vi "test_read-nmea-data2.vi"() -> ()   [LabVIEW 2019] (continued)
A,3,85,70,71,84,,,,,,,,,1.18,0.66,0.97,2*04\n\t\n15:14:01.34\tF9P\t$GNGSA,A,3,36,19,11,04,09,12,,,,,,,1.18,0.66,0.97,3*06\n\t\n15:14:01.36\tF9P\t$GNGSA,A,3,14,11,33,,,,,,,,,,1.18,0.66,0.97,4*07\n\t\n15:14:01.38\tF9P\t$GPGSV,3,1,09,02,55,320,27,04,17,043,32,05,38,248,30,06,64,050,27,1*6A\n\t\n15:14:01.40\tF9P\t$GPGSV,3,2,09,09,44,073,35,12,23,276,23,17,32,154,33,19,51,157,29,1*64\n\t\n15:14:01.42\tF9P\t$GPGSV,3,3,09,25,12,306,16,1*5B\n\t\n15:14:01.44\tF9P\t$GPGSV,3,1,09,02,55,320,,04,17,043,21,05,38,248,17,06,64,050,24,6*6C\n\t\n15:14:01.46\tF9P\t$GPGSV,3,2,09,09,44,073,29,12,23,276,13,17,32,154,19,19,51,157,,6*6E\n\t\n15:14:01.48\tF9P\t$GPGSV,3,3,09,25,12,306,,6*5B\n\t\n15:14:01.50\tF9P\t$GLGSV,2,1,08,69,11,031,34,70,70,038,25,71,53,206,26,72,05,210,,1*76\n\t\n15:14:01.52\tF9P\t$GLGSV,2,2,08,77,01,325,,84,19,123,17,85,70,070,29,86,37,330,,1*7B\n\t\n15:14:01.54\tF9P\t$GLGSV,2,1,08,69,11,031,29,70,70,038,,71,53,206,23,72,05,210,,3*7A\n\t\n15:14:01.56\tF9P\t$GLGSV,2,2,08,77,01,325,,84,19,123,23,85,70,070,22,86,37,330,,3*75\n\t\n15:14:01.58\tF9P\t$GAGSV,2,1,08,02,08,296,16,04,67,115,35,09,33,193,22,11,72,001,24,7*7E\n\t\n15:14:01.60\tF9P\t$GAGSV,2,2,08,12,39,103,24,19,25,045,22,25,09,249,,36,26,308,10,7*72\n\t\n15:14:01.62\tF9P\t$GAGSV,2,1,08,02,08,296,,04,67,115,26,09,33,193,,11,72,001,,2*78\n\t\n15:14:01.64\tF9P\t$GAGSV,2,2,08,12,39,103,,19,25,045,,25,09,249,,36,26,308,,2*70\n\t\n15:14:01.66\tF9P\t$GBGSV,1,1,04,11,49,132,27,14,87,114,32,28,,,30,33,61,220,33,1*4B\n\t\n15:14:01.68\tF9P\t$GBGSV,1,1,04,08,,,36,11,49,132,26,14,87,114,28,33,61,220,,3*47\n\t\n15:14:01.70\tF9P\t$GNGLL,3723.58118,N,12656.98443,E,061403.00,A,A*73\n\t\n15:14:01.72\tF9P\t\t\n15:14:01.74\tF9P\t\t\n15:14:01.76\tF9P\t\t\n15:14:01.78\tF9P\t\t\n15:14:01.80\tF9P\t\t\n15:14:01.82\tF9P\t\t\n15:14:01.84\tF9P\t\t\n15:14:01.86\tF9P\t\t\n15:14:01.88\tF9P\t\t\n15:14:01.90\tF9P\t\t\n15:14:01.92\tF9P\t\t\n15:14:01.94\tF9P\t\t\n15:14:01.96\tF9P\t\t\n15:14:01.98\tF9P\t\t\n15:14:02.00\tF9P\t\t\n15:14:02.02\tF9P\t\t\n15:14:02.04\tF9P\t\t\n15:14:02.06\tF9P\t\t\n15:14:02.08\tF9P\t\t\n15:14:02.10\tF9P\t\t\n15:14:02.12\tF9P\t\t\n15:14:02.14\tF9P\t\t\n15:14:02.16\tF9P\t\t\n15:14:02.18\tF9P\t\t\n15:14:02.20\tF9P\t\t\n15:14:02.22\tF9P\t\t\n15:14:02.24\tF9P\t$GNRMC,061404.00,A,3723.58195,N,12656.98403,E,2.222,333.91,250720,,,A,V*01\n\t\n15:14:02.26\tF9P\t$GNVTG,333.91,T,,M,2.222,N,4.115,K,A*29\n\t\n15:14:02.28\tF9P\t$GNGGA,061404.00,3723.58195,N,12656.98403,E,1,12,0.71,48.3,M,18.5,M,,*76\n\t\n15:14:02.30\tF9P\t$GNGSA,A,3,12,06,19,05,17,09,04,02,,,,,1.27,0.71,1.05,1*06\n\t\n15:14:02.32\tF9P\t$GNGSA,A,3,85,70,71,84,,,,,,,,,1.27,0.71,1.05,2*04\n\t\n15:14:02.34\tF9P\t$GNGSA,A,3,36,19,11,04,09,12,,,,,,,1.27,0.71,1.05,3*06\n\t\n15:14:02.36\tF9P\t$GNGSA,A,3,14,11,33,,,,,,,,,,1.27,0.71,1.05,4*07\n\t\n15:14:02.38\tF9P\t$GPGSV,3,1,09,02,55,320,31,04,17,043,35,05,38,248,36,06,64,050,28,1*63\n\t\n15:14:02.40\tF9P\t$GPGSV,3,2,09,09,44,073,35,12,23,276,22,17,32,154,39,19,51,157,33,1*64\n\t\n15:14:02.42\tF9P\t$GPGSV,3,3,09,25,12,306,14,1*59\n\t\n15:14:02.44\tF9P\t$GPGSV,3,1,09,02,55,320,,04,17,043,21,05,38,248,20,06,64,050,23,6*6F\n\t\n15:14:02.46\tF9P\t$GPGSV,3,2,09,09,44,073,21,12,23,276,10,17,32,154,19,19,51,157,,6*65\n\t\n15:14:02.48\tF9P\t$GPGSV,3,3,09,25,12,306,,6*5B\n\t\n15:14:02.50\tF9P\t$GLGSV,2,1,08,69,11,031,34,70,70,038,23,71,53,206,31,72,05,210,,1*76\n\t\n15:14:02.52\tF9P\t$GLGSV,2,2,08,77,01,325,,84,19,123,19,85,70,070,24,86,37,330,,1*78\n\t\n15:14:02.54\tF9P\t$GLGSV,2,1,08,69,11,031,29,70,70,038,,71,53,206,29,72,05,210,,3*70\n\t\n15:14:02.56\tF9P\t$GLGSV,2,2,08,77,01,325,,84,19,123,30,85,70,070,21,86,37,330,,3*74\n\t\n15:14:02.58\tF9P\t$GAGSV,2,1,08,02,08,296,10,04,67,115,32,09,33,193,23,11,72,001,25,7*7F\n\t\n15:14:02.60\tF9P\t$GAGSV,2,2,08,12,39,103,34,19,25,045,30,25,09,249,,36,26,308,13,7*73\n\t\n15:14:02.62\tF9P\t$GAGSV,2,1,08,02,08,296,,04,67,115,32,09,33,193,,11,72,001,,2*7D\n\t\n15:14:02.64\tF9P\t$GAGSV,2,2,08,12,39,103,,19,25,045,,25,09,249,,36,26,308,,2*70\n\t\n15:14:02.66\tF9P\t$GBGSV,1,1,04,11,49,132,33,14,87,114,29,28,,,29,33,61,220,37,1*48\n\t\n15:14:02.68\tF9P\t$GBGSV,1,1,04,08,,,27,11,49,132,29,14,87,114,28,33,61,220,,3*48\n\t\n15:14:02.70\tF9P\t$GNGLL,3723.58195,N,12656.98403,E,061404.00,A,A*75\n\t\n15:14:02.72\tF9P\t\t\n15:14:02.74\tF9P\t\t\n15:14:02.76\tF9P\t\t\n15:14:02.78\tF9P\t\t\n15:14:02.80\tF9P\t\t\n15:14:02.82\tF9P\t\t\n15:14:02.84\tF9P\t\t\n15:14:02.86\tF9P\t\t\n15:14:02.88\tF9P\t\t\n15:14:02.90\tF9P\t\t\n15:14:02.92\tF9P\t\t\n15:14:02.94\tF9P\t\t\n15:14:02.96\tF9P\t\t\n15:14:02.98\tF9P\t\t\n15:14:03.00\tF9P\t\t\n15:14:03.02\tF9P\t\t\n15:14:03.04\tF9P\t\t\n15:14:03.06\tF9P\t\t\n15:14:03.08\tF9P\t\t\n15:14:03.10\tF9P\t\t\n15:14:03.12\tF9P\t\t\n15:14:03.14\tF9P\t\t\n15:14:03.16\tF9P\t\t\n15:14:03.18\tF9P\t\t\n15:14:03.20\tF9P\t\t\n15:14:03.22\tF9P\t\t\n15:14:03.24\tF9P\t$GNRMC,061405.00,A,3723.58265,N,12656.98422,E,1.873,346.43,250720,,,A,V*0F\n\t\n15:14:03.26\tF9P\t$GNVTG,346.43,T,,M,1.873,N,3.469,K,A*20\n\t\n15:14:03.28\tF9P\t$GNGGA,061405.00,3723.58265,N,12656.98422,E,1,12,0.71,47.7,M,18.5,M,,*73\n\t\n15:14:03.30\tF9P\t$GNGSA,A,3,12,06,19,05,17,09,04,02,,,,,1.27,0.71,1.05,1*06\n\t\n15:14:03.32\tF9P\t$GNGSA,A,3,85,70,71,84,,,,,,,,,1.27,0.71,1.05,2*04\n\t\n15:14:03.34\tF9P\t$GNGSA,A,3,36,19,11,04,09,12,,,,,,,1.27,0.71,1.05,3*06\n\t\n15:14:03.36\tF9P\t$GNGSA,A,3,14,11,33,,,,,,,,,,1.27,0.71,1.05,4*07\n\t\n15:14:03.38\tF9P\t$GPGSV,3,1,09,02,55,320,31,04,17,043,32,05,38,248,26,06,64,050,36,1*6A\n\t\n15:14:03.40\tF9P\t$GPGSV,3,2,09,09,44,073,40,12,23,276,21,17,32,154,33,19,51,157,32,1*6E\n\t\n15:14:03.42\tF9P\t$GPGSV,3,3,09,25,12,306,10,1*5D\n\t\n15:14:03.44\tF9P\t$GPGSV,3,1,09,02,55,320,,04,17,043,29,05,38,248,21,06,64,050,29,6*6C\n\t\n15:14:03.46\tF9P\t$GPGSV,3,2,09,09,44,073,30,12,23,276,,17,32,154,21,19,51,157,,6*6F\n\t\n15:14:03.48\tF9P\t$GPGSV,3,3,09,25,12,306,,6*5B\n\t\n15:14:03.50\tF9P\t$GLGSV,2,1,08,69,11,031,35,70,70,038,21,71,53,206,39,72,05,210,,1*7D\n\t\n15:14:03.52\tF9P\t$GLGSV,2,2,08,77,01,325,,84,19,123,29,85,70,070,29,86,37,330,,1*76\n\t\n15:14:03.54\tF9P\t$GLGSV,2,1,08,69,11,031,22,70,70,038,,71,53,206,29,72,05,210,,3*7B\n\t\n15:14:03.56\tF9P\t$GLGSV,2,2,08,77,01,325,,84,19,123,29,85,70,070,21,86,37,330,,3*7C\n\t\n15:14:03.58\tF9P\t$GAGSV,2,1,08,02,08,296,16,04,67,115,29,09,33,193,22,11,72,001,26,7*71\n\t\n15:14:03.60\tF9P\t$GAGSV,2,2,08,12,39,103,29,19,25,045,29,25,08,248,,36,26,308,14,7*70\n\t\n15:14:03.62\tF9P\t$GAGSV,2,1,08,02,08,296,,04,67,115,25,09,33,193,,11,72,001,,2*7B\n\t\n15:14:03.64\tF9P\t$GAGSV,2,2,08,12,39,103,,19,25,045,,25,08,248,,36,26,308,,2*70\n\t\n15:14:03.66\tF9P\t$GBGSV,1,1,04,11,49,132,31,14,87,114,30,28,,,33,33,61,220,29,1*46\n\t\n15:14:03.68\tF9P\t$GBGSV,1,1,04,08,,,28,11,49,132,38,14,87,114,33,33,61,220,,3*4D\n\t\n15:14:03.70\tF9P\t$GNGLL,3723.58265,N,12656.98422,E,061405.00,A,A*7B\n\t\n15:14:03.72\tF9P\t\t\n15:14:03.74\tF9P\t\t\n15:14:03.76\tF9P\t\t\n15:14:03.78\tF9P\t\t\n15:14:03.80\tF9P\t\t\n15:14:03.82\tF9P\t\t\n15:14:03.84\tF9P\t\t\n15:14:03.86\tF9P\t\t\n15:14:03.88\tF9P\t\t\n15:14:03.90\tF9P\t\t\n15:14:03.92\tF9P\t\t\n15:14:03.94\tF9P\t\t\n15:14:03.96\tF9P\t\t\n15:14:03.98\tF9P\t\t\n15:14:04.00\tF9P\t\t\n15:14:04.02\tF9P\t\t\n15:14:04.04\tF9P\t\t\n15:14:04.06\tF9P\t\t\n15:14:04.08\tF9P\t\t\n15:14:04.10\tF9P\t\t\n15:14:04.12\tF9P\t\t\n15:14:04.14\tF9P\t\t\n15:14:04.16\tF9P\t\t\n15:14:04.18\tF9P\t\t\n15:14:04.20\tF9P\t\t\n15:14:04.22\tF9P\t\t\n15:14:04.24\tF9P\t$GNRMC,061406.00,A,3723.58360,N,12656.98387,E,2.422,350.86,250720,,,A,V*05\n\t\n15:14:04.26\tF9P\t$GNVTG,350.86,T,,M,2.422,N,4.486,K,A*23\n\t\n15:14:04.28\tF9P\t$GNGGA,061406.00,3723.58360,N,12656.98387,E,1,12,0.71,47.4,M,18.5,M,,*7F\n\t\n15:14:04.30\tF9P\t$GNGSA,A,3,12,06,19,05,17,09,04,02,,,,,1.27,0.71,1.05,1*06\n\t\n15:14:04.32\tF9P\t$GNGSA,A,3,85,70,71,84,,,,,,,,,1.27,0.71,1.05,2*04\n\t\n15:14:04.34\tF9P\t$GNGSA,A,3,36,19,11,04,09,12,,,,,,,1.27,0.71,1.05,3*06\n\t\n15:14:04.36\tF9P\t$GNGSA,A,3,14,11,33,,,,,,,,,,1.27,0.71,1.05,4*07\n\t\n15:14:04.38\tF9P\t$GPGSV,3,1,09,02,55,320,29,04,17,043,31,05,38,248,37,06,64,050,29,1*6E\n\t\n15:14:04.40\tF9P\t$GPGSV,3,2,09,09,44,073,31,12,23,276,20,17,32,154,41,19,51,157,30,1*6E\n\t\n15:14:04.42\tF9P\t$GPGSV,3,3,09,25,12,306,12,1*5F\n\t\n15:14:04.44\tF9P\t$GPGSV,3,1,09,02,55,320,,04,17,043,24,05,38,248,20,06,64,050,28,6*61\n\t\n15:14:04.46\tF9P\t$GPGSV,3,2,09,09,44,073,23,12,23,276,,17,32,154,22,19,51,157,,6*6E\n\t\n15:14:04.48\tF9P\t$GPGSV,3,3,09,25,12,306,,6*5B\n\t\n15:14:04.50\tF9P\t$GLGSV,2,1,08,69,11,031,34,70,70,038,23,71,53,206,31,72,05,210,,1*76\n\t\n15:14:04.52\tF9P\t$GLGSV,2,2,08,77,01,325,,84,19,123,29,85,70,070,33,86,37,330,,1*7D\n\t\n15:14:04.54\tF9P\t$GLGSV,2,1,08,69,11,031,24,70,70,038,,71,53,206,23,72,05,210,,3*77\n\t\n15:14:04.56\tF9P\t$GLGSV,2,2,08,77,01,325,,84,19,123,24,85,70,070,22,86,37,330,,3*72\n\t\n15:14:04.58\tF9P\t$GAGSV,2,1,08,02,08,296,14,04,67,115,29,09,33,193,22,11,72,001,26,7*73\n\t\n15:14:04.60\tF9P\t$GAGSV,2,2,08,12,39,103,33,19,25,045,29,25,08,248,,36,26,308,13,7*7C\n\t\n15:14:04.62\tF9P\t$GAGSV,2,1,08,02,08,296,,04,67,115,,09,33,193,,11,72,001,,2*7C\n\t\n15:14:04.64\tF9P\t$GAGSV,2,2,08,12,39,103,,19,25,045,,25,08,248,,36,26,308,,2*70\n\t\n15:14:04.66\tF9P\t$GBGSV,1,1,04,11,49,132,36,14,87,114,34,28,,,30,33,61,220,36,1*48\n\t\n15:14:04.68\tF9P\t$GBGSV,1,1,04,08,,,28,11,49,132,32,14,87,114,32,33,61,220,,3*46\n\t\n15:14:04.70\tF9P\t$GNGLL,3723.58360,N,12656.98387,E,061406.00,A,A*74\n\t\n15:14:04.72\tF9P\t\t\n15:14:04.74\tF9P\t\t\n15:14:04.76\tF9P\t\t\n15:14:04.78\tF9P\t\t\n15:14:04.80\tF9P\t\t\n15:14:04.82\tF9P\t\t\n15:14:04.84\tF9P\t\t\n15:14:04.86\tF9P\t\t\n15:14:04.88\tF9P\t\t\n15:14:04.90\tF9P\t\t\n15:14:04.92\tF9P\t\t\n15:14:04.94\tF9P\t\t\n15:14:04.96\tF9P\t\t\n15:14:04.98\tF9P\t\t\n15:14:05.00\tF9P\t\t\n15:14:05.02\tF9P\t\t\n15:14:05.04\tF9P\t\t\n15:14:05.06\tF9P\t\t\n15:14:05.08\tF9P\t\t\n15:14:05.10\tF9P\t\t\n15:14:05.12\tF9P\t\t\n15:14:05.14\tF9P\t\t\n15:14:05.16\tF9P\t\t\n15:14:05.18\tF9P\t\t\n15:14:05.20\tF9P\t\t\n15:14:05.22\tF9P\t\t\n15:14:05.24\tF9P\t$GNRMC,061407.00,A,3723.58436,N,12656.98343,E,1.577,346.00,250720,,,A,V*03\n\t\n15:14:05.26\tF9P\t$GNVTG,346.00,T,,M,1.577,N,2.920,K,A*2F\n\t\n15:14:05.28\tF9P\t$GNGGA,061407.00,3723.58436,N,12656.98343,E,1,12,0.71,45.6,M,18.5,M,,*72\n\t\n15:14:05.30\tF9P\t$GNGSA,A,3,12,06,19,05,17,09,04,02,,,,,1.27,0.71,1.05,1*06\n\t\n15:14:05.32\tF9P\t$GNGSA,A,3,85,70,71,84,,,,,,,,,1.27,0.71,1.05,2*04\n\t\n15:14:05.34\tF9P\t$GNGSA,A,3,36,19,11,04,09,12,,,,,,,1.27,0.71,1.05,3*06\n\t\n15:14:05.36\tF9P\t$GNGSA,A,3,14,11,33,,,,,,,,,,1.27,0.71,1.05,4*07\n\t\n15:14:05.38\tF9P\t$GPGSV,3,1,09,02,55,320,33,04,17,043,27,05,38,248,32,06,64,050,30,1*6F\n\t\n15:14:05.40\tF9P\t$GPGSV,3,2,09,09,44,073,32,12,23,276,21,17,32,154,37,19,51,157,33,1*6E\n\t\n15:14:05.42\tF9P\t$GPGSV,3,3,09,25,12,306,16,1*5B\n\t\n15:14:05.44\tF9P\t$GPGSV,3,1,09,02,55,320,,04,17,043,23,05,38,248,21,06,64,050,25,6*6A\n\t\n15:14:05.46\tF9P\t$GPGSV,3,2,09,09,44,073,24,12,23,276,,17,32,154,21,19,51,157,,6*6A\n\t\n15:14:05.48\tF9P\t$GPGSV,3,3,09,25,12,306,,6*5B\n\t\n15:14:05.50\tF9P\t$GLGSV,2,1,08,69,11,031,37,70,70,038,22,71,53,206,33,72,05,210,,1*76\n\t\n15:14:05.52\tF9P\t$GLGSV,2,2,08,77,01,325,,84,19,123,32,85,70,070,28,86,37,330,,1*7D\n\t\n15:14:05.54\tF9P\t$GLGSV,2,1,08,69,11,031,25,70,70,038,,71,53,206,23,72,05,210,,3*76\n\t\n15:14:05.56\tF9P\t$GLGSV,2,2,08,77,01,325,,84,19,123,30,85,70,070,22,86,37,330,,3*77\n\t\n15:14:05.58\tF9P\t$GAGSV,2,1,08,02,08,296,16,04,67,115,29,09,33,193,21,11,72,001,25,7*71\n\t\n15:14:05.60\tF9P\t$GAGSV,2,2,08,12,39,103,29,19,25,045,27,25,08,248,,36,26,308,15,7*7F\n\t\n15:14:05.62\tF9P\t$GAGSV,2,1,08,02,08,296,,04,67,115,,09,33,193,,11,72,001,,2*7C\n\t\n15:14:05.64\tF9P\t$GAGSV,2,2,08,12,39,103,,19,25,045,,25,08,248,,36,26,308,,2*70\n\t\n15:14:05.66\tF9P\t$GBGSV,1,1,04,11,49,132,32,14,87,114,30,28,,,30,33,61,220,38,1*46\n\t\n15:14:05.68\tF9P\t$GBGSV,1,1,04,08,,,29,11,49,132,28,14,87,114,33,33,61,220,,3*4D\n\t\n15:14:05.70\tF9P\t$GNGLL,3723.58436,N,12656.98343,E,061407.00,A,A*79\n\t\n15:14:05.72\tF9P\t\t\n15:14:05.74\tF9P\t\t\n15:14:05.76\tF9P\t\t\n15:14:05.78\tF9P\t\t\n15:14:05.80\tF9P\t\t\n15:14:05.82\tF9P\t\t\n15:14:05.84\tF9P\t\t\n15:14:05.86\tF9P\t\t\n15:14:05.88\tF9P\t\t\n15:14:05.90\tF9P\t\t\n15:14:05.92\tF9P\t\t\n15:14:05.94\tF9P\t\t\n15:14:05.96\tF9P\t\t\n15:14:05.98\tF9P\t\t\n15:14:06.00\tF9P\t\t\n15:14:06.02\tF9P\t\t\n15:14:06.04\tF9P\t\t\n15:14:06.06\tF9P\t\t\n15:14:06.08\tF9P\t\t\n15:14:06.10\tF9P\t\t\n15:14:06.12\tF9P\t\t\n15:14:06.14\tF9P\t\t\n15:14:06.16\tF9P\t\t\n15:14:06.18\tF9P\t\t\n15:14:06.20\tF9P\t\t\n15:14:06.22\tF9P\t\t\n15:14:06.24\tF9P\t$GNRMC,061408.00,A,3723.58491,N,12656.98325,E,1.921,339.14,250720,,,A,V*03\n\t\n15:14:06.26\tF9P\t$GNVTG,339.14,T,,M,1.921,N,3.558,K,A*2F\n\t\n15:14:06.28\tF9P\t$GNGGA,061408.00,3723.58491,N,12656.98325,E,1,12,0.71,46.3,M,18.5,M,,*76\n\t\n15:14:06.30\tF9P\t$GNGSA,A,3,12,06,19,05,17,09,04,02,,,,,1.27,0.71,1.05,1*06\n\t\n15:14:06.32\tF9P\t$GNGSA,A,3,85,70,71,84,,,,,,,,,1.27,0.71,1.05,2*04\n\t\n15:14:06.34\tF9P\t$GNGSA,A,3,36,19,11,04,09,12,,,,,,,1.27,0.71,1.05,3*06\n\t\n15:14:06.36\tF9P\t$GNGSA,A,3,14,11,33,,,,,,,,,,1.27,0.71,1.05,4*07\n\t\n15:14:06.38\tF9P\t$GPGSV,3,1,09,02,55,320,32,04,17,043,31,05,38,248,29,06,64,050,30,1*63\n\t\n15:14:06.40\tF9P\t$GPGSV,3,2,09,09,44,073,27,12,23,276,22,17,32,154,37,19,51,157,25,1*6E\n\t\n15:14:06.42\tF9P\t$GPGSV,3,3,09,25,12,306,17,1*5A\n\t\n15:14:06.44\tF9P\t$GPGSV,3,1,09,02,55,320,,04,17,043,24,05,38,248,21,06,64,050,23,6*6B\n\t\n15:14:06.46\tF9P\t$GPGSV,3,2,09,09,44,073,31,12,23,276,,17,32,154,22,19,51,157,,6*6D\n\t\n15:14:06.48\tF9P\t$GPGSV,3,3,09,25,12,306,,6*5B\n\t\n15:14:06.50\tF9P\t$GLGSV,2,1,08,69,11,031,33,70,70,038,23,71,53,206,38,72,05,210,,1*78\n\t\n15:14:06.52\tF9P\t$GLGSV,2,2,08,77,01,325,,84,19,123,30,85,70,070,27,86,37,330,,1*70\n\t\n15:14:06.54\tF9P\t$GLGSV,2,1,08,69,11,031,25,70,70,038,,71,53,206,35,72,05,210,,3*71\n\t\n15:14:06.56\tF9P\t$GLGSV,2,2,08,77,01,325,,84,19,123,30,85,70,070,20,86,37,330,,3*75\n\t\n15:14:06.58\tF9P\t$GAGSV,2,1,08,02,08,296,09,04,67,115,33,09,33,193,22,11,72,001,25,7*77\n\t\n15:14:06.60\tF9P\t$GAGSV,2,2,08,12,39,103,31,19,25,045,27,25,08,248,,36,26,308,18,7*7B\n\t\n15:14:06.62\tF9P\t$GAGSV,2,1,08,02,08,296,,04,67,115,,09,33,193,,11,72,001,,2*7C\n\t\n15:14:06.64\tF9P\t$GAGSV,2,2,08,12,39,103,,19,25,045,,25,08,248,,36,26,308,,2*70\n\t\n15:14:06.66\tF9P\t$GBGSV,1,1,04,11,49,132,26,14,87,114,30,28,,,25,33,61,220,40,1*48\n\t\n15:14:06.68\tF9P\t$GBGSV,1,1,04,08,,,28,11,49,132,28,14,87,114,25,33,61,220,,3*4B\n\t\n15:14:06.70\tF9P\t$GNGLL,3723.58491,N,12656.98325,E,061408.00,A,A*7B\n\t\n15:14:06.72\tF9P\t\t\n15:14:06.74\tF9P\t\t\n15:14:06.76\tF9P\t\t\n15:14:06.78\tF9P\t\t\n15:14:06.80\tF9P\t\t\n15:14:06.82\tF9P\t\t\n15:14:06.84\tF9P\t\t\n15:14:06.86\tF9P\t\t\n15:14:06.88\tF9P\t\t\n15:14:06.90\tF9P\t\t\n15:14:06.92\tF9P\t\t\n15:14:06.94\tF9P\t\t\n15:14:06.96\tF9P\t\t\n15:14:06.98\tF9P\t\t\n15:14:07.00\tF9P\t\t\n15:14:07.02\tF9P\t\t\n15:14:07.04\tF9P\t\t\n15:14:07.06\tF9P\t\t\n15:14:07.08\tF9P\t\t\n15:14:07.10\tF9P\t\t\n15:14:07.12\tF9P\t\t\n15:14:07.14\tF9P\t\t\n15:14:07.16\tF9P\t\t\n15:14:07.18\tF9P\t\t\n15:14:07.20\tF9P\t\t\n15:14:07.22\tF9P\t\t\n15:14:07.24\tF9P\t$GNRMC,061409.00,A,3723.58569,N,12656.98296,E,2.411,341.14,250720,,,A,V*0F\n\t\n15:14:07.26\tF9P\t$GNVTG,341.14,T,,M,2.411,N,4.466,K,A*26\n\t\n15:14:07.28\tF9P\t$GNGGA,061409.00,3723.58569,N,12656.98296,E,1,12,0.71,46.0,M,18.5,M,,*7B\n\t\n15:14:07.30\tF9P\t$GNGSA,A,3,12,06,19,05,17,09,04,02,,,,,1.27,0.71,1.05,1*06\n\t\n15:14:07.32\tF9P\t$GNGSA,A,3,85,70,71,84,,,,,,,,,1.27,0.71,1.05,2*04\n\t\n15:14:07.34\tF9P\t$GNGSA,A,3,36,19,11,04,09,12,,,,,,,1.27,0.71,1.05,3*06\n\t\n15:14:07.36\tF9P\t$GNGSA,A,3,14,11,33,,,,,,,,,,1.27,0.71,1.05,4*07\n\t\n15:14:07.38\tF9P\t$GPGSV,3,1,09,02,55,320,27,04,17,043,26,05,38,248,27,06,64,050,29,1*67\n\t\n15:14:07.40\tF9P\t$GPGSV,3,2,09,09,44,073,26,12,23,276,24,17,32,154,34,19,51,157,29,1*66\n\t\n15:14:07.42\tF9P\t$GPGSV,3,3,09,25,12,306,16,1*5B\n\t\n15:14:07.44\tF9P\t$GPGSV,3,1,09,02,55,320,,04,17,043,22,05,38,248,19,06,64,050,22,6*67\n\t\n15:14:07.46\tF9P\t$GPGSV,3,2,09,09,44,073,26,12,23,276,,17,32,154,22,19,51,157,,6*6B\n\t\n15:14:07.48\tF9P\t$GPGSV,3,3,09,25,12,306,,6*5B\n\t\n15:14:07.50\tF9P\t$GLGSV,2,1,08,69,11,031,29,70,70,038,22,71,53,206,40,72,05,210,,1*7D\n\t\n15:14:07.52\tF9P\t$GLGSV,2,2,08,77,01,325,,84,19,123,30,85,70,070,26,86,37,330,,1*71\n\t\n15:14:07.54\tF9P\t$GLGSV,2,1,08,69,11,031,24,70,70,038,,71,53,206,31,72,05,210,,3*74\n\t\n15:14:07.56\tF9P\t$GLGSV,2,2,08,77,01,325,,84,19,123,34,85,70,070,18,86,37,330,,3*7A\n\t\n15:14:07.58\tF9P\t$GAGSV,2,1,08,02,08,296,11,04,67,115,28,09,33,193,23,11,72,001,26,7*76\n\t\n15:14:07.60\tF9P\t$GAGSV,2,2,08,12,39,103,30,19,25,045,27,25,08,248,,36,26,308,10,7*72\n\t\n15:14:07.62\tF9P\t$GAGSV,2,1,08,02,08,296,,04,67,115,,09,33,193,,11,72,001,,2*7C\n\t\n15:14:07.64\tF9P\t$GAGSV,2,2,08,12,39,103,,19,25,045,,25,08,248,,36,26,308,,2*70\n\t\n15:14:07.66\tF9P\t$GBGSV,1,1,04,11,49,132,28,14,87,114,28,28,,,25,33,61,220,37,1*4F\n\t\n15:14:07.68\tF9P\t$GBGSV,1,1,04,08,,,30,11,49,132,,14,87,114,,33,61,220,,3*4F\n\t\n15:14:07.70\tF9P\t$GNGLL,3723.58569,N,12656.98296,E,061409.00,A,A*75\n\t\n15:14:07.72\tF9P\t\t\n15:14:07.74\tF9P\t\t\n15:14:07.76\tF9P\t\t\n15:14:07.78\tF9P\t\t\n15:14:07.80\tF9P\t\t\n15:14:07.82\tF9P\t\t\n15:14:07.84\tF9P\t\t\n15:14:07.86\tF9P\t\t\n15:14:07.88\tF9P\t\t\n15:14:07.90\tF9P\t\t\n15:14:07.92\tF9P\t\t\n15:14:07.94\tF9P\t\t\n15:14:07.96\tF9P\t\t\n15:14:07.98\tF9P\t\t\n15:14:08.00\tF9P\t\t\n15:14:08.02\tF9P\t\t\n15:14:08.04\tF9P\t\t\n15:14:08.06\tF9P\t\t\n15:14:08.08\tF9P\t\t\n15:14:08.10\tF9P\t\t\n15:14:08.12\tF9P\t\t\n15:14:08.14\tF9P\t\t\n15:14:08.16\tF9P\t\t\n15:14:08.18\tF9P\t\t\n15:14:08.20\tF9P\t\t\n15:14:08.22\tF9P\t\t\n15:14:08.24\tF9P\t$GNRMC,061410.00,A,3723.58634,N,12656.98260,E,2.145,337.68,250720,,,A,V*0B\n\t\n15:14:08.26\tF9P\t$GNVTG,337.68,T,,M,2.145,N,3.973,K,A*26\n\t\n15:14:08.28\tF9P\t$GNGGA,061410.00,3723.58634,N,12656.98260,E,1,12,0.71,46.2,M,18.5,M,,*73\n\t\n15:14:08.30\tF9P\t$GNGSA,A,3,12,06,19,05,17,09,04,02,,,,,1.27,0.71,1.05,1*06\n\t\n15:14:08.32\tF9P\t$GNGSA,A,3,85,70,71,84,,,,,,,,,1.27,0.71,1.05,2*04\n\t\n15:14:08.34\tF9P\t$GNGSA,A,3,36,19,11,04,09,12,,,,,,,1.27,0.71,1.05,3*06\n\t\n15:14:08.36\tF9P\t$GNGSA,A,3,14,11,33,,,,,,,,,,1.27,0.71,1.05,4*07\n\t\n15:14:08.38\tF9P\t$GPGSV,3,1,09,02,55,320,26,04,17,043,26,05,38,248,35,06,64,050,34,1*69\n\t\n15:14:08.40\tF9P\t$GPGSV,3,2,09,09,44,073,27,12,23,276,24,17,32,154,33,19,51,157,33,1*6B\n\t\n15:14:08.42\tF9P\t$GPGSV,3,3,09,25,12,306,17,1*5A\n\t\n15:14:08.44\tF9P\t$GPGSV,3,1,09,02,55,320,,04,17,043,20,05,38,248,21,06,64,050,23,6*6F\n\t\n15:14:08.46\tF9P\t$GPGSV,3,2,09,09,44,073,27,12,23,276,,17,32,154,22,19,51,157,,6*6A\n\t\n15:14:08.48\tF9P\t$GPGSV,3,3,09,25,12,306,,6*5B\n\t\n15:14:08.50\tF9P\t$GLGSV,2,1,08,69,11,031,32,70,70,038,24,71,53,206,38,72,05,210,,1*7E\n\t\n15:14:08.52\tF9P\t$GLGSV,2,2,08,77,01,325,,84,19,123,28,85,70,070,34,86,37,330,,1*7B\n\t\n15:14:08.54\tF9P\t$GLGSV,2,1,08,69,11,031,24,70,70,038,,71,53,206,25,72,05,210,,3*71\n\t\n15:14:08.56\tF9P\t$GLGSV,2,2,08,77,01,325,,84,19,123,30,85,70,070,20,86,37,330,,3*75\n\t\n15:14:08.58\tF9P\t$GAGSV,2,1,08,02,08,296,12,04,67,115,28,09,33,193,24,11,72,001,25,7*71\n\t\n15:14:08.60\tF9P\t$GAGSV,2,2,08,12,39,103,30,19,25,045,26,25,08,248,,36,26,308,10,7*73\n\t\n15:14:08.62\tF9P\t$GAGSV,2,1,08,02,08,296,,04,67,115,,09,33,193,,11,72,001,,2*7C\n\t\n15:14:08.64\tF9P\t$GAGSV,2,2,08,12,39,103,,19,25,045,,25,08,248,,36,26,308,,2*70\n\t\n15:14:08.66\tF9P\t$GBGSV,1,1,04,11,49,132,27,14,87,114,32,28,,,32,33,61,220,36,1*4C\n\t\n15:14:08.68\tF9P\t$GBGSV,1,1,03,11,49,132,29,14,87,114,,33,61,220,,3*48\n\t\n15:14:08.70\tF9P\t$GNGLL,3723.58634,N,12656.98260,E,061410.00,A,A*7F\n\t\n15:14:08.72\tF9P\t\t\n15:14:08.74\tF9P\t\t\n15:14:08.76\tF9P\t\t\n15:14:08.78\tF9P\t\t\n15:14:08.80\tF9P\t\t\n15:14:08.82\tF9P\t\t\n15:14:08.84\tF9P\t\t\n15:14:08.86\tF9P\t\t\n15:14:08.88\tF9P\t\t\n15:14:08.90\tF9P\t\t\n15:14:08.92\tF9P\t\t\n15:14:08.94\tF9P\t\t\n15:14:08.96\t
